vi "数据处理直接插入整合 (子VI).vi"   [LabVIEW 2016, in "数据传输系统.lvlib"]
types:
  T1 = cluster{"PH":string[][], "CODCr":string[][], "氨氮":string[][], "CODMn":string[][], "总氮":string[][], "总磷":string[][], "电导率":string[][], "水温":string[][], "DO":string[][], "浊度":string[][], "叶绿素":string[][], "藻密度":string[][], "铜":string[][], "盐度":string[][], "水位":string[][], "流速":string[][], "瞬时流量":string[][], "累积流量":string[][], "亚硝酸盐":string[][], "硫化物":string[][], "ORP":string[][]}
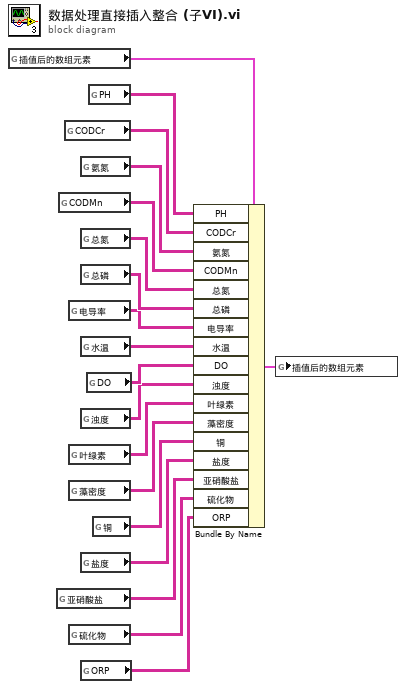
[diagram p0: block diagram]
diagram:
  n1 = global read "插值后的新数组.vi" "插值后的数组元素"() -> (w5:T1)
  n2 = global read "全局 所有参数.vi" "亚硝酸盐"() -> (w2:string[][])
  n3 = global read "全局 所有参数.vi" "CODMn"() -> (w16:string[][])
  n4 = global read "全局 所有参数.vi" "CODCr"() -> (w18:string[][])
  n5 = global read "全局 所有参数.vi" "电导率"() -> (w13:string[][])
  n6 = global read "全局 所有参数.vi" "叶绿素"() -> (w9:string[][])
  n7 = global read "全局 所有参数.vi" "藻密度"() -> (w8:string[][])
  n8 = global read "全局 所有参数.vi" "硫化物"() -> (w3:string[][])
  n9 = global read "全局 所有参数.vi" "氨氮"() -> (w17:string[][])
  n10 = global read "全局 所有参数.vi" "总氮"() -> (w15:string[][])
  n11 = global read "全局 所有参数.vi" "总磷"() -> (w14:string[][])
  n12 = global read "全局 所有参数.vi" "水温"() -> (w12:string[][])
  n13 = global read "全局 所有参数.vi" "浊度"() -> (w10:string[][])
  n14 = global read "全局 所有参数.vi" "盐度"() -> (w6:string[][])
  n15 = global read "全局 所有参数.vi" "ORP"() -> (w4:string[][])
  n16 = global read "全局 所有参数.vi" "DO"() -> (w11:string[][])
  n17 = global read "全局 所有参数.vi" "PH"() -> (w19:string[][])
  n18 = global read "全局 所有参数.vi" "铜"() -> (w7:string[][])
  n19 = Bundle By Name(cluster=w5, "PH"=w19, "CODCr"=w18, "氨氮"=w17, "CODMn"=w16, "总氮"=w15, "总磷"=w14, "电导率"=w13, "水温"=w12, "DO"=w11, "浊度"=w10, "叶绿素"=w9, "藻密度"=w8, "铜"=w7, "盐度"=w6, "亚硝酸盐"=w2, "硫化物"=w3, "ORP"=w4) -> (w1:T1)
  n20 = global write "插值后的新数组.vi" "插值后的数组元素"(w1) -> ()
